vi "Handling Published Globals.vi"() -> ()   [LabVIEW 2015]
uses:
  Handling Operations.ctl
panel:
  in  "Median Speed of Shooter":dbl=40.0
  in  "Shooter Output Speed":dbl
  in  "Handler Operation":T1
  # "Tip: The global is a good way publish state or\ninformational/debugging values.\nIt is not  advised that you put setpoint values here."
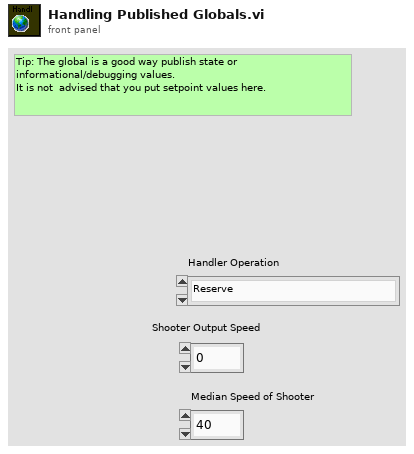
[diagram p1: front panel]
types:
  T1 = typedef "Handling Operations.ctl" = enum16{"Reserve", "Read Current", "Pickup Ball", "Fire", "Fire at Setspeed"}
diagram:
